vi "libconnected.vi"(8 "error in (no error)":errorcluster, 11 "input":i32) -> (0 "error out":errorcluster, 2 "connected":bool)   [LabVIEW 2015]
uses:
  <vilib>/Utility/error.llb/DialogType.ctl
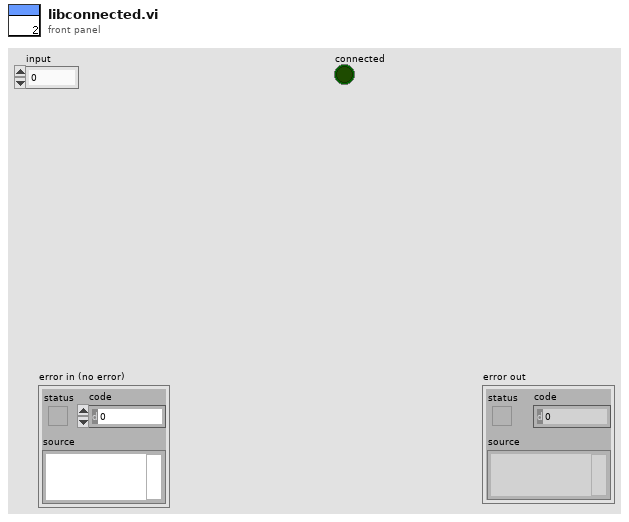
[diagram p1: front panel]
types:
  T1 = typedef "DialogType.ctl" = u16
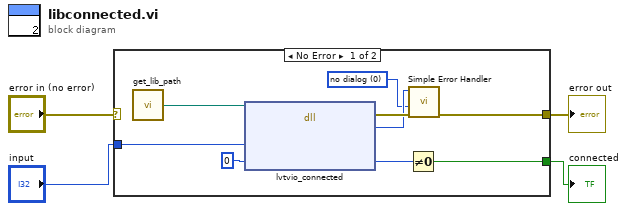
[diagram p0: block diagram]
diagram:
  n1 = case shown="No Error" "error in (no error)" {
    selector: "error in (no error)" -> [_ w14]
    tunnel: [w11 w14] -> w3
    tunnel: [w6 _] -> w2
    tunnel: "input" -> [w5 _]
    frame No Error {
      w7 = T1 0 items=["no dialog", "OK message", "continue or stop message", "OK message + warnings", "continue/stop + warnings"] ("type of dialog (OK msg:1)")
      n2 = call "get_lib_path.vi"() -> ("Path"=w13:path)
      n3 = dll-call lib="S:/thingiverselv/lib/liblvtvio.dll" fn="lvtvio_connected"(path in=w13, "input"=w5, "is"=0) -> (error out=w12:errorcluster, "return type"=w10:i32, "is"=w8:i32)  [unwired: 3 in, 1 out]
      n4 = Not Equal To 0?(x=w8) -> (x != 0?=w6:bool)
      n5 = call <vilib>:"Simple Error Handler.vi"("error code (no error:0)"=w10, "type of dialog (OK msg:1)"=w7, "error in (no error)"=w12) -> ("error out"=w11:errorcluster)  [unwired: 2 in, 4 out]
    }
    frame Error {
    }
  }
  "error out" <- w3
  "connected" <- w2
